vi "Get MB Channel by Name.vi"(8 "error in (no error)":errorcluster, 9 "Active Line Name":string, 11 "Modbus Module configuration in":refnum<class "Modbus Module configuration.lvclass">) -> (0 "error out":errorcluster, 1 "index":i32, 2 "Modbus Module Channel.lvclass":refnum<class "Modbus Module Channel.lvclass">, 3 "Modbus Module configuration out":refnum<class "Modbus Module configuration.lvclass">)   [LabVIEW 2013, in "Modbus Module editor node.lvclass"]
uses:
  Modbus Module editor node.lvclass
  module/module channel/Modbus Module Channel.lvclass
  module/configuration/Modbus Module configuration.lvclass
  <vilib>/NI/Tag Bus/tag/tag descriptor.lvclass
  <vilib>/NI/Tag Bus/tag/tag descriptor.lvclass/tag descriptor.ctl
  <vilib>/NI/Tag Bus/tag/read tag name.vi
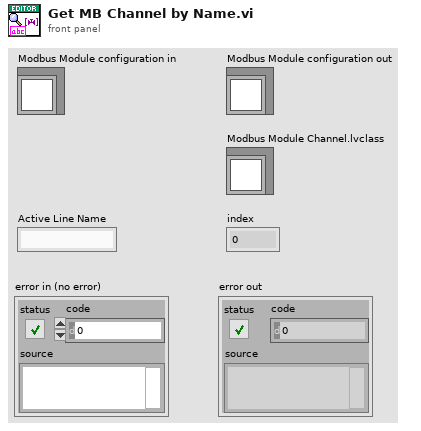
[diagram p1: front panel]
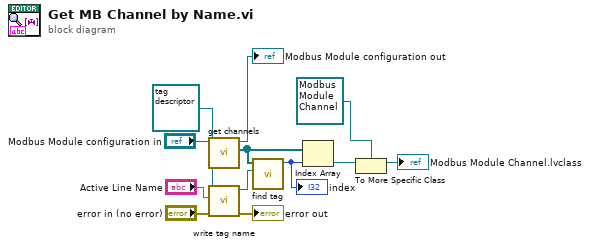
[diagram p0: block diagram]
diagram:
  n1 = call-dynamic "get channels.vi"("Modbus Slave configuration in"="Modbus Module configuration in") -> ("channels"=w5:refnum<class "TBM channel.lvclass">[], "Modbus Slave configuration out"=→"Modbus Module configuration out":refnum<class "Modbus Module configuration.lvclass">)  [unwired: 9 in]
  n2 = call <vilib>:"write tag name.vi"("error in"="error in (no error)", "name"="Active Line Name", "system tag in"=refnum<class "tag descriptor.lvclass"> refnum) -> ("error out"=→"error out":errorcluster, "system tag out"=w6:refnum<class "tag descriptor.lvclass">)  [unwired: 7 in]
  n3 = call <vilib>:"find tag.vi"("tag"=w6, "tags in"=w5) -> ("index"=w8:i32)  [unwired: 9 in]
  "index" <- w8
  n4 = Index Array(array=w5, index=w8) -> (element=w11:refnum<class "TBM channel.lvclass">)
  n5 = To More Specific Class(target class=refnum<class "Modbus Module Channel.lvclass"> refnum ("Modbus Module Channel.lvclass"), reference=w11) -> (specific class reference=→"Modbus Module Channel.lvclass":refnum<class "Modbus Module Channel.lvclass">)  [unwired: 1 in, 1 out]
